vi "Clear.vi"(3 "(WavBuf)":refnum<class "(WavBuf).lvclass">) -> (1 "(WavBuf) Out":refnum<class "(WavBuf).lvclass">)   [LabVIEW 2016, in "(WavBuf).lvclass"]
uses:
  (WavBuf).lvclass
  (WavBuf).lvclass/(WavBuf).ctl
  Universal Controls/Read Write Button.ctl
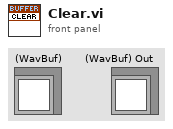
[diagram p1: front panel]
types:
  T1 = typedef "Read Write Button.ctl" = bool
  T2 = typedef "Ref_DVR_Buffer.ctl" = refnum<data-value>
  T3 = typedef "Waveform_Data.ctl" = waveform(dbl)
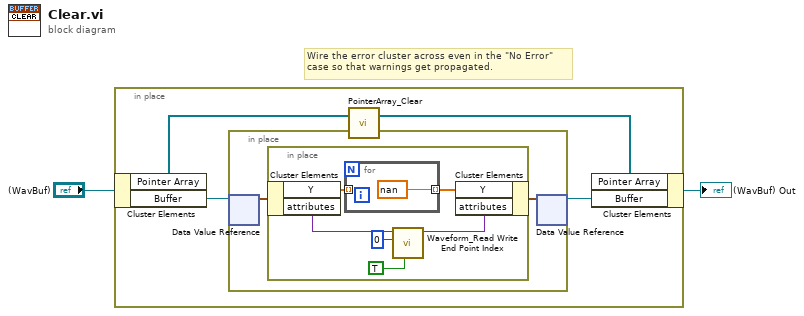
[diagram p0: block diagram]
diagram:
  # "Wire the error cluster across even in the \"No Error\"\ncase so that warnings get propagated."
  n1 = in-place {
    n2 = in-place-cluster #1("(WavBuf)") -> ("Pointer Array"=w6:refnum<class "((Pointer)).lvclass">[], "Buffer"=w4:T2)
    n3 = in-place {
      n4 = in-place-dvr #2(w4) -> (w8:T3)  [unwired: 1 out]
      n5 = in-place {
        n6 = in-place-cluster #3(w8) -> ("Y"=w14:dbl[], "attributes"=w12:variant)
        n7 = for {
          tunnel: w14 -> [_] mode=indexing
          tunnel: [nan] -> w13 mode=indexing
        }
        n8 = call "Waveform_Read Write End Point Index.vi"("Read(f)\nWrite(t)"=T1 TRUE ("Read(f)\nWrite(t)"), "End Point"=0, "Waveform Atributes"=w12) -> ("Waveform Atributes Out"=w11:variant)  [unwired: 6 in, 2 out]
        n9 = in-place-cluster #3("Y"=w13, "attributes"=w11) -> (w7:T3)
      }
      n10 = in-place-dvr #2(w7) -> (w3:T2)  [unwired: 1 out]
    }
    n11 = call "PointerArray_Clear.vi"("Pointer Array"=w6) -> ("Pointer Array Out"=w5:refnum<class "((Pointer)).lvclass">[])  [unwired: 2 in]
    n12 = in-place-cluster #1("Pointer Array"=w5, "Buffer"=w3) -> (→"(WavBuf) Out":refnum<class "(WavBuf).lvclass">)
  }
